vi "Construct Child.vi"(8 "error in (no error)":errorcluster, 9 "Ignored":bool, 10 "Offset":dbl) -> (0 "error out":errorcluster, 3 "Child out":refnum<class "Child.lvclass">)   [LabVIEW 2017, in "Composition.Tests.lvlib" / "Child.lvclass"]
uses:
  Child.lvclass
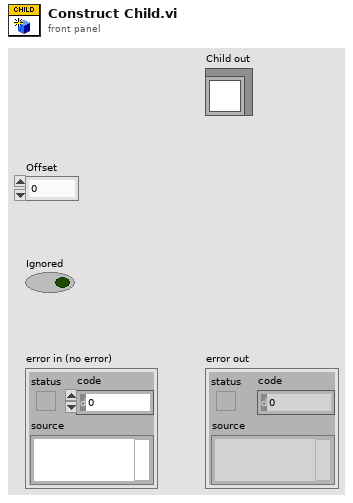
[diagram p1: front panel]
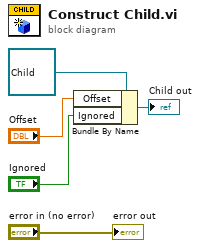
[diagram p0: block diagram]
diagram:
  n1 = Bundle By Name(cluster=refnum<class "Child.lvclass"> refnum ("Child in"), "Offset"="Offset", "Ignored"="Ignored") -> (→"Child out":refnum<class "Child.lvclass">)
  "error out" <- "error in (no error)"
